vi "2DLev-Mar xx.vi"(1 "W":dbl[](array[numeric]) format="%.2f", 2 "Function":refnum<vi>, 3 "error":i32, 4 "Coefficients":dbl[](array[numeric]) format="%.2f", 5 "Y":dbl[](array[numeric]) format="%.2f", 6 "X":dbl[](array[numeric]) format="%.2f") -> (0 "chiSqr":dbl format="%.2f")   [LabVIEW 2016]
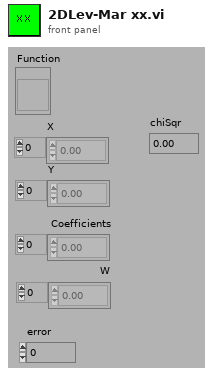
[diagram p1: front panel]
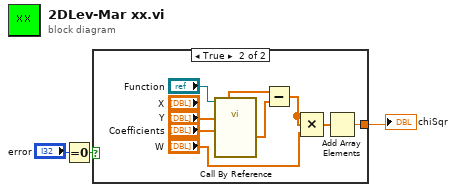
[diagram p0: block diagram]
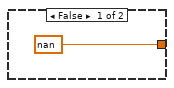
[diagram p2: hidden frame]
diagram:
  n1 = Equal To 0?(x="error") -> (x = 0?=w2:bool)
  n2 = case shown="True" w2 {
    tunnel: [nan w10] -> w1
    frame False {
    }
    frame True {
      n3 = call-by-ref "?"(reference="Function", "Paramters"="Coefficients") -> ("Simulated Image"=w6:dbl[])  [unwired: 1 in, 2 out]
      n4 = Subtract(x="Y", y=w6) -> (x-y=w11:dbl[])
      n5 = Compound Arithmetic op=MULTIPLY(w11, w11, "W") -> (w9:dbl[])
      n6 = Add Array Elements(numeric array=w9) -> (sum=w10:dbl)
    }
  }
  "chiSqr" <- w1
